vi "Write Waveform.vi"(4 "CIC filter factor":dbl=4.0 format="%#_13g", 6 "Input scale":dbl=1.0 format="%#_6p", 8 "error in (no error)":errorcluster, 10 "I-V parameters":T2={"Start magnitude"=0.001, "Magnitude increment"=0.001, "End magnitude"=0.01, "Ramp length"=0, "Top  length"=0, "Threshold "=2e-06, "Processing delay"=0, "Output gain "=0.001, "Interpolation"=64, "Stop after"=1, "Detector window"=480} {"Detector window" format="%dpts"; "Stop after" format="%d sweep(s)"; "Output gain" format="%#_6pA/V"; "Processing delay" format="%dpts"; "Threshold" format="%#_6pV"; "Top  length" format="%dpts"; "Ramp length" format="%dpts"; "End magnitude" format="%#_6pA"; "Magnitude increment" format="%#_6pA"; "Start magnitude" format="%#_6pA"}, 11 "RP Communicator in":refnum<class "RP Communicator.lvclass">) -> (0 "error out":errorcluster, 2 "Output Waveform":i16[](graph), 3 "RP Communicator out":refnum<class "RP Communicator.lvclass">)   [LabVIEW 2024, in "RP Communicator.lvclass"]
uses:
  RP Communicator.lvclass
  Waform generation/I-V parameters.ctl
  RP EEPROM Calibration.ctl
  RP Communicator.lvclass/RP Communicator.ctl
  Read RP EEPROM Calibration.vi
panel:
  out "RP EEPROM Calib":T1 {"magic" format="%x"}
  in  "RP EEPROM Calibration":T1={"In1 LV scale"=50254123, "In2 LV scale"=50320266, "In1 HV scale"=987584779, "In2 HV scale"=988813140, "In1 HV offset"=-58, "In2 HV offset"=-73, "Out1 scale"=47310353, "Out2 scale"=47421163, "Out1 offset"=-107, "Out2 offset"=-98, "magic"=2864434397, "In1 LV offset"=-71, "In2 LV offset"=-89} {"magic" format="%x"}
  # "Waveform parameters"
  # "Detector parameters"
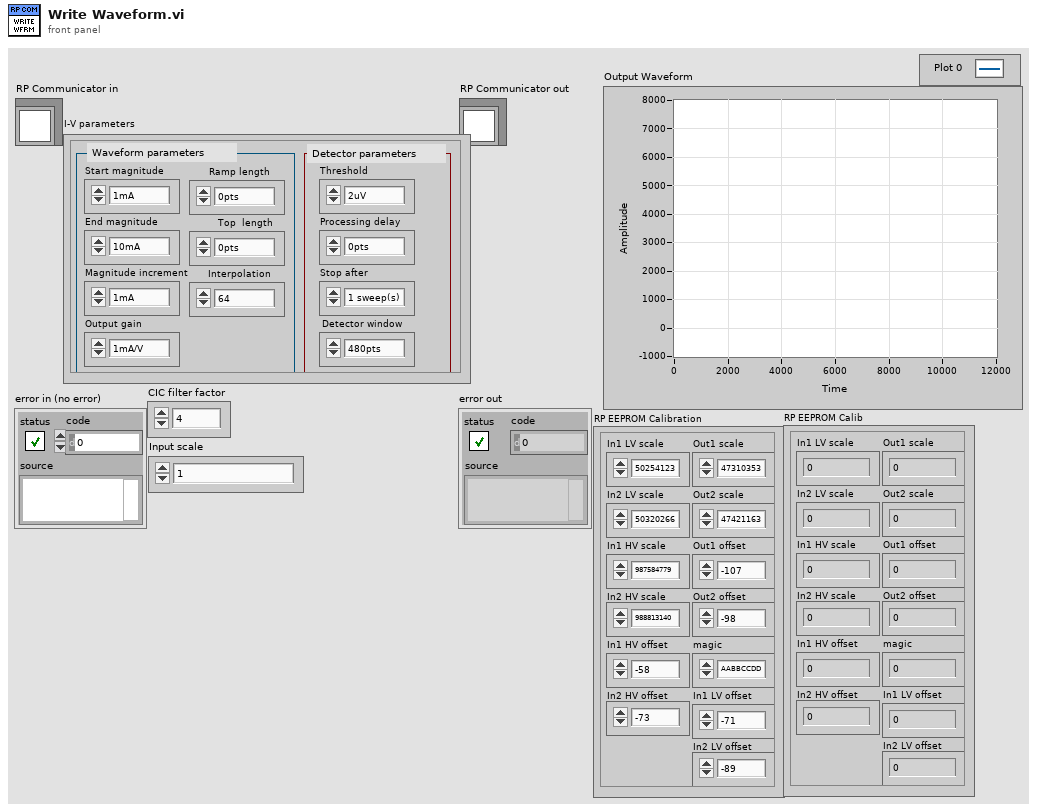
[diagram p1: front panel]
types:
  T1 = typedef "RP EEPROM Calibration.ctl" = cluster{"In1 LV scale":u32, "In2 LV scale":u32, "In1 HV scale":u32, "In2 HV scale":u32, "In1 HV offset":i32, "In2 HV offset":i32, "Out1 scale":u32, "Out2 scale":u32, "Out1 offset":i32, "Out2 offset":i32, "magic":u32, "In1 LV offset":i32, "In2 LV offset":i32}
  T2 = typedef "I-V parameters.ctl" = cluster{"Start magnitude":dbl, "Magnitude increment":dbl, "End magnitude":dbl, "Ramp length":i32, "Top  length":i32, "Threshold ":dbl, "Processing delay":u16, "Output gain ":dbl, "Interpolation":i32, "Stop after":u16, "Detector window":i32}
  T3 = enum16{"big-endian, network order", "native, host order", "little-endian"}
  T4 = typedef "Waveform parameters.ctl" = cluster{"Start magnitude":dbl, "Magnitude increment":dbl, "Number of pulses":i32, "Ramp length":i32, "Top  length":i32, "Threshold ":i32, "Processing delay":u16, "Stop after":u16, "Detector window":i32, "Upper limit":i16, "Lower limit":i16}
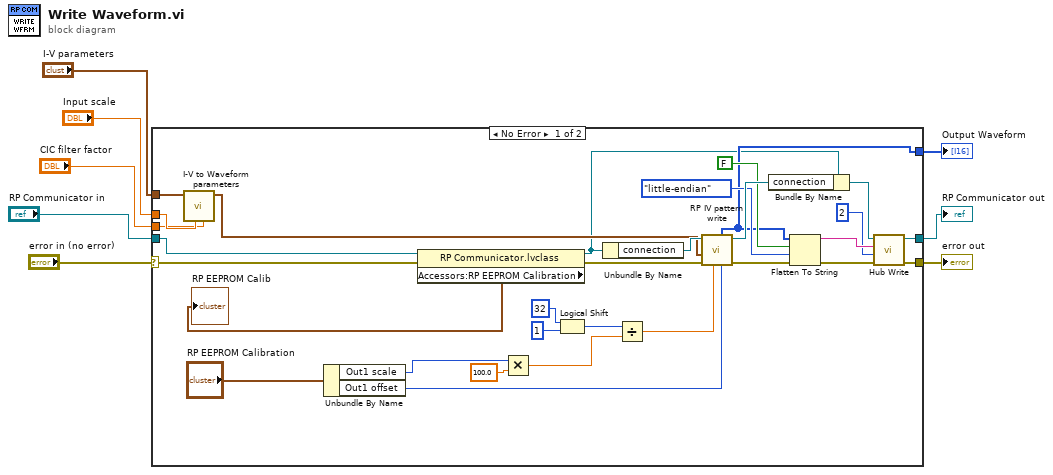
[diagram p0: block diagram]
diagram:
  n1 = case shown="No Error" "error in (no error)" {
    selector: "error in (no error)" -> [w35 w40]
    tunnel: [w30 w40] -> w7
    tunnel: [w31 w39] -> w5
    tunnel: "RP Communicator in" -> [w20 w39]
    tunnel: "I-V parameters" -> [w38 _]
    tunnel: [w26 _] -> w3
    tunnel: "CIC filter factor" -> [w32 _]
    tunnel: "Input scale" -> [w33 _]
    frame No Error {
      n2 = call "I-V to Waveform parameters.vi"("CIC filter factor"=w32, "Input scale"=w33, "I-V parameters"=w38) -> ("Waveform parameters out"=w36:T4)  [unwired: 8 in]
      n3 = Unbundle By Name("RP EEPROM Calibration") -> ("Out1 scale"=w13:u32, "Out1 offset"=w9:i32)
      n4 = property class="RP Communicator.lvclass"(reference=w20, error in=w35) -> (reference out=w19:refnum<class "RP Communicator.lvclass">, error out=w21:errorcluster, "Accessors:RP EEPROM Calibration"=→"RP EEPROM Calib":T1)
      n5 = Multiply(x=w13, y=100.0) -> (x*y=w11:dbl)
      n6 = Logical Shift(y=i16 32, x=u64 1) -> (x << y=w12:u64)
      n7 = Unbundle By Name(w19) -> ("connection"=w37:refnum<k5>)
      n8 = Divide(x=w12, y=w11) -> (x/y=w10:dbl)
      n9 = call "RP IV pattern write.vi"("Out offset"=w9, "Out scale"=w10, "Error In"=w21, "Waveform parameters"=w36, "connection ID"=w37) -> ("Error Out"=w25:errorcluster, "connection ID out"=w34:refnum<k5>, "Waveform Graph"=w26:i16[])  [unwired: 4 in]
      n10 = Bundle By Name(cluster=w19, "connection"=w34) -> (w29:refnum<class "RP Communicator.lvclass">)
      n11 = Flatten To String(anything=w26, prepend array or string size? (T)=FALSE, byte order (0:big-endian, network order)=T3."little-endian", error in (no error)=w25) -> (data string=w23:string, error out=w24:errorcluster)  [unwired: 1 out]
      n12 = call-dynamic "Hub Write.vi"("error in (no error)"=w24, "hub port"=u64 2, "data in"=w23, "RP Communicator in"=w29) -> ("error out"=w30:errorcluster, "RP Communicator out"=w31:refnum<class "RP Communicator.lvclass">)  [unwired: 6 in]
    }
    frame Error {
    }
  }
  "error out" <- w7
  "RP Communicator out" <- w5
  "Output Waveform" <- w3
